vi "pelletizing pyton test.vi"() -> ()   [LabVIEW 2019]
uses:
  detectedPellet.lvlib
panel:
  out "Image 3":T1(plugin-control)
  out "Image":T1(plugin-control)
  in  "img path":path
  out "error out":errorcluster
  in  "module path":path
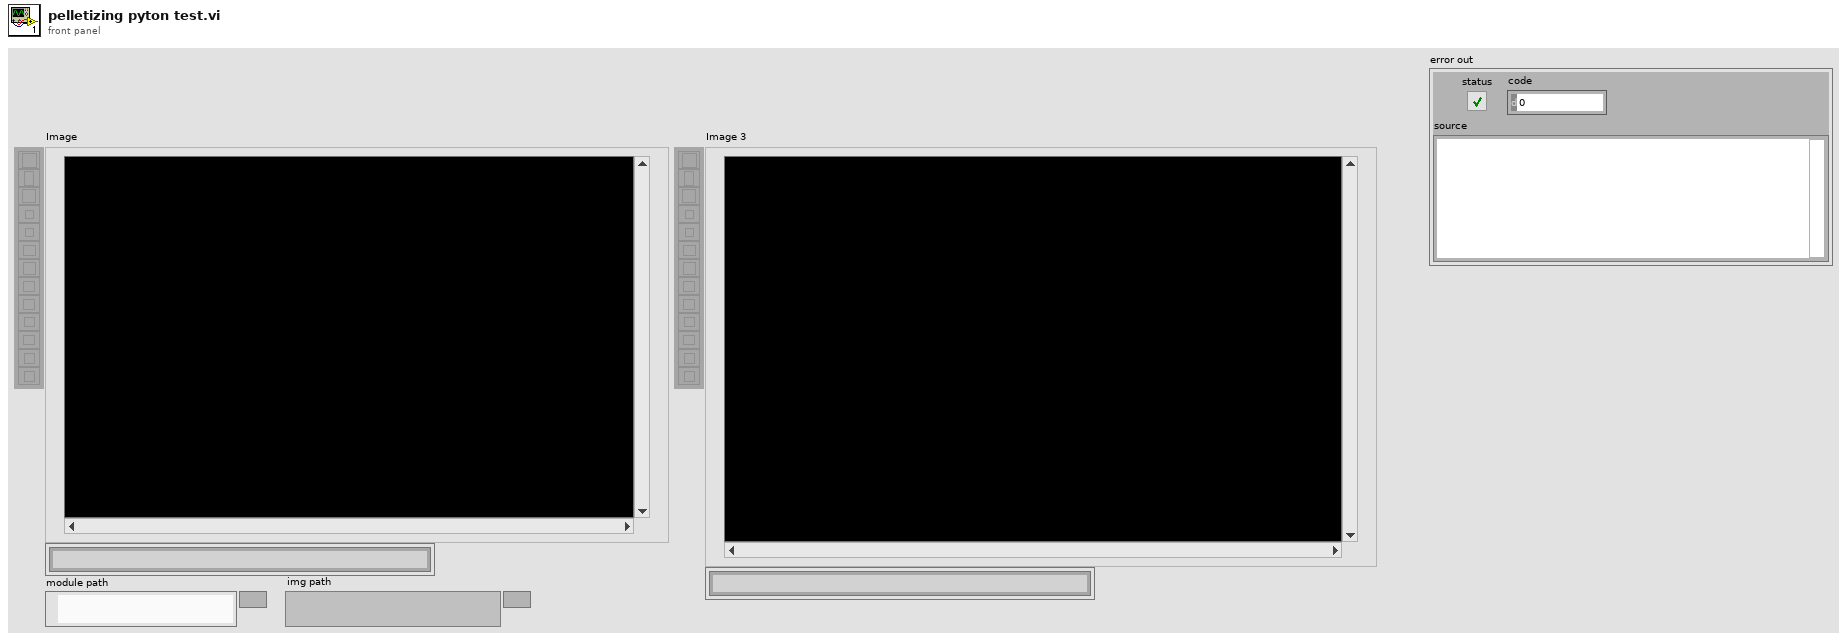
[diagram p1: front panel]
types:
  T1 = typedef "IMAQ Image.ctl" = refnum<image>
  T2 = typedef "Image Type" = u32
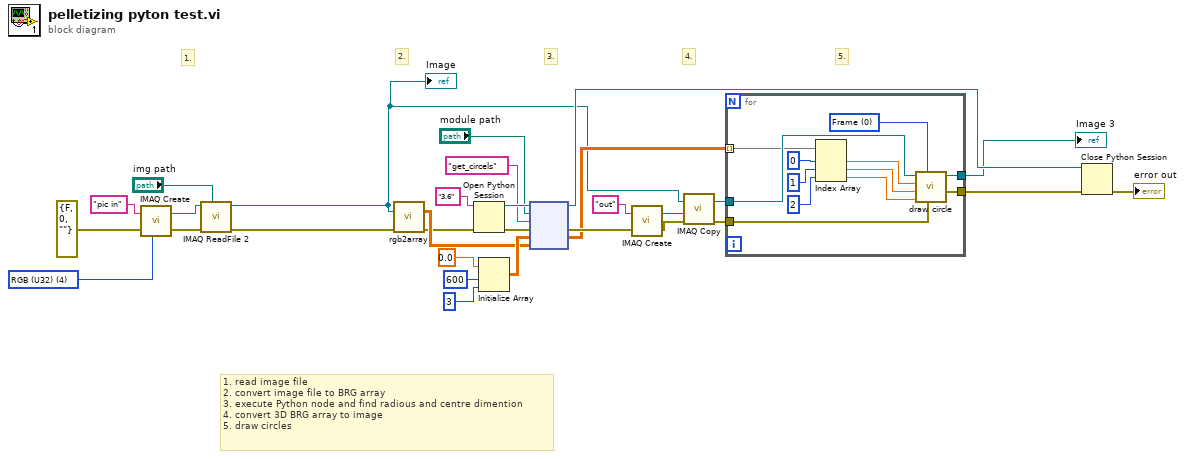
[diagram p0: block diagram]
diagram:
  w26 = T2 4 items=["Grayscale (U8)", "Grayscale (I16)", "Grayscale (SGL)", "Complex (CSG)", "RGB (U32)", "HSL (U32)", "RGB (U64)", "Grayscale (U16)"] ("Image Type")
  # "1. read image file\n2. convert image file to BRG array\n3. execute Python node and find radious and centre dimention\n4. convert 3D BRG array to image\n5. draw circles"
  # "5."
  # "4."
  # "3."
  # "2."
  # "1."
  n1 = call "IMAQ Create"("Image Name"="pic in", "Image Type"=w26, "error in (no error)"=errorcluster {"status"=FALSE, "code"=0, "source"=""}) -> ("New Image"=w27:T1, "error out"=w28:errorcluster)  [unwired: 2 in]
  n2 = call "IMAQ ReadFile 2"("File Path"="img path", "error in (no error)"=w28, "Image"=w27) -> ("error out"=w5:errorcluster, "Image Out"=w1:T1)  [unwired: 4 in, 3 out]
  "Image" <- w1
  n3 = call "rgb2array.vi"("Image IN"=w1, "error in (no error)"=w5) -> ("output Array"=w4:dbl[][][], "error out"=w3:errorcluster)  [unwired: 12 in]
  n4 = Open Python Session(python version="3.6" ("Python version"), 3:w3) -> (session out=w21:refnum<k35>, error out=w22:errorcluster)  [unwired: 1 in]
  n5 = Initialize Array(0.0 ("element"), 600 ("dimension size"), 3 ("dimension size")) -> (w14:dbl[][])
  n6 = node(w21, "module path", "get_circels" ("function name"), w22, w14, w4) -> (w18:refnum<k35>, w12:errorcluster, w6:dbl[][])  [unwired: 1 in, 2 out]
  n7 = call "IMAQ Create"("Image Name"="out", "error in (no error)"=w12) -> ("New Image"=w11:T1, "error out"=w2:errorcluster)  [unwired: 3 in]
  n8 = call "IMAQ Copy"("error in (no error)"=w2, "Image Dst"=w11, "Image Src"=w1) -> ("error out"=w9:errorcluster, "Image Dst Out"=w10:T1)  [unwired: 3 in]
  n9 = for {
    tunnel: w10 -> [w42]
    tunnel: w6 -> [w41] mode=indexing
    tunnel: w9 -> [w33]
    tunnel: [w32] -> w8
    tunnel: [w31] -> w7
    w34 = u32 0 items=["Frame", "Fill"] ("Drawing Mode (Frame)")
    n10 = Index Array(array=w41, index #1=0 ("index"), index #2=1 ("index"), index #3=2 ("index")) -> (element #1=w37:dbl, element #2=w36:dbl, element #3=w35:dbl)
    n11 = call "draw circle.vi"("error in (no error)"=w33, "Drawing Mode (Frame)"=w34, "box size"=w35, "Y"=w36, "X"=w37, "Image In"=w42) -> ("error out"=w32:errorcluster, "Image Out"=w31:T1)  [unwired: 4 in]
  }
  "Image 3" <- w7
  n12 = Close Python Session(session in=w18, error in=w8) -> (11:→"error out":errorcluster)
